vi "Get MIDI files.vi"(8 "error in (no error)":errorcluster) -> (0 "error out":errorcluster, 3 "Available MIDI Files":string[](array[string]))   [LabVIEW 2016]
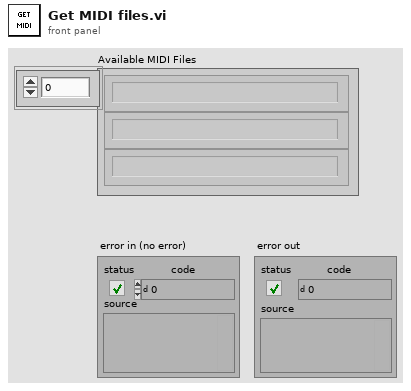
[diagram p1: front panel]
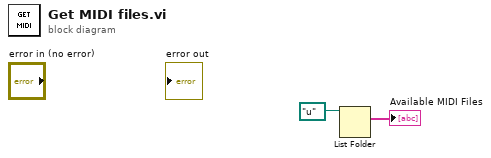
[diagram p0: block diagram]
diagram:
  n1 = List Folder(path=path "u:/" ("selected path")) -> (filenames=→"Available MIDI Files":string[])  [unwired: 3 in, 3 out]
